vi "ns1970.vi"() -> (1 "ns1970":u64)   [LabVIEW 2025, in "MdfFile.lvlib"]
uses:
  MdfFile.lvlib
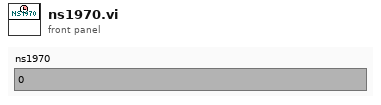
[diagram p1: front panel]
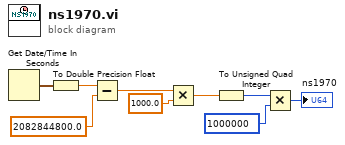
[diagram p0: block diagram]
diagram:
  n1 = Get Date/Time In Seconds() -> (seconds since 1Jan1904=w3:timestamp)
  n2 = To Double Precision Float(number=w3) -> (double precision float=w9:dbl)
  n3 = Subtract(x=w9, y=2082844800.0) -> (x-y=w1:dbl)
  n4 = Multiply(x=w1, y=1000.0) -> (x*y=w2:dbl)
  n5 = To Unsigned Quad Integer(1:w2) -> (0:w6:u64)
  n6 = Multiply(x=w6, y=u64 1000000) -> (x*y=→"ns1970":u64)
